vi "写入数据.vi"(7 "工作表名称":string="Sheet1", 8 "错误输入（无错误）":errorcluster, 9 "数据":variant, 10 "单元格区域":T2, 11 "引用簇":T1) -> (0 "错误输出":errorcluster, 3 "引用簇输出":T1)   [LabVIEW 2021, in "OperateExcel.lvlib"]
uses:
  OperateExcel.lvlib
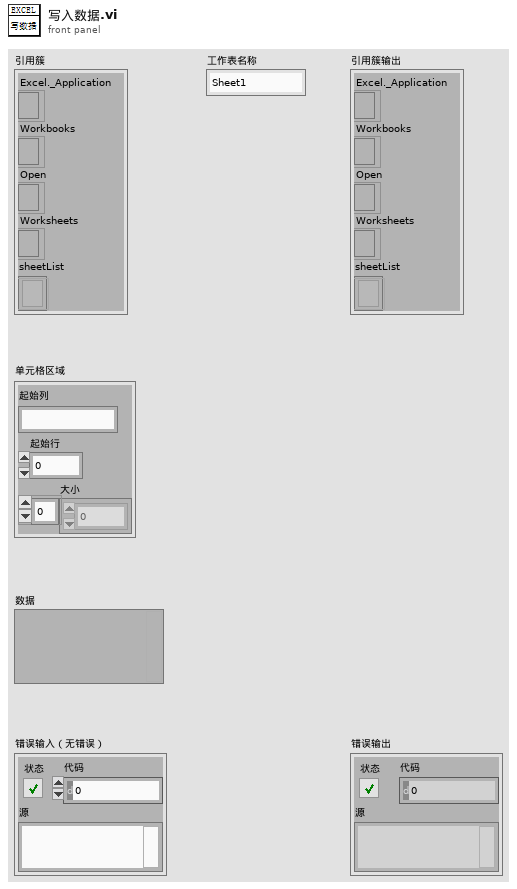
[diagram p1: front panel]
types:
  T1 = typedef "OperateExcel.lvlib/引用簇.ctl" = cluster{"Excel._Application":refnum<k7>, "Workbooks":refnum<k7>, "Open":refnum<k7>, "Worksheets":refnum<k7>, "sheetList":refnum<k7>[]}
  T2 = typedef "OperateExcel.lvlib/单元格区域.ctl" = cluster{"起始列":string, "起始行":i32, "大小":i32[]}
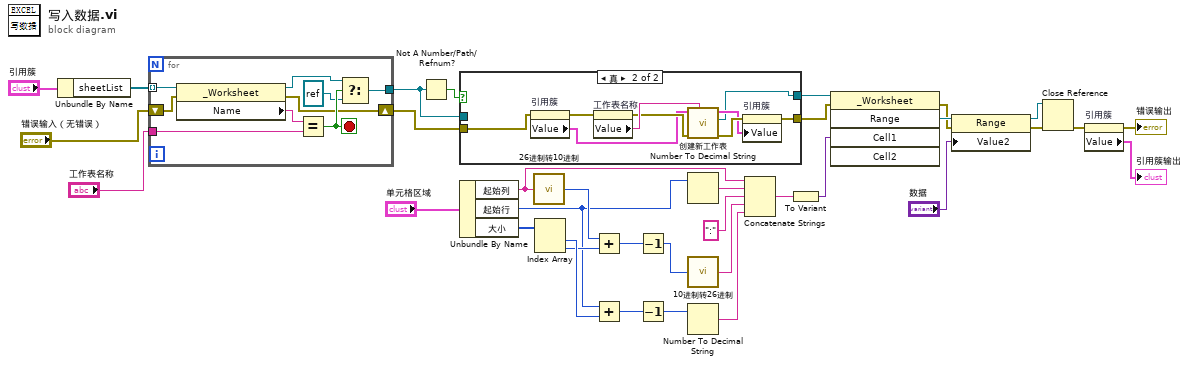
[diagram p0: block diagram]
diagram:
  n1 = Unbundle By Name("引用簇") -> ("sheetList"=w34:refnum<k7>[])
  n2 = for {
    tunnel: w34 -> [w43] mode=indexing
    tunnel: "工作表名称" -> [w41]
    tunnel: [w37] -> w31
    shift-right: [w35] -> w28
    shift-left: "错误输入（无错误）" -> [w36]
    stop <- w40 stop-if-true
    n3 = property class="_Worksheet"(reference=w43, error in=w36) -> (reference out=w38:refnum<k7>, error out=w35:errorcluster, "Name"=w42:string)
    n4 = Equal?(x=w42, y=w41) -> (x = y?=w40:bool)
    n5 = Select(t=w38, s=w40, f=refnum<k7> refnum ("自动化引用句柄")) -> (s? t:f=w37:refnum<k7>)
  }
  n6 = Not A Number/Path/Refnum?(number/path/refnum=w31) -> (NaN/Path/Refnum?=w32:bool)
  n7 = case shown="真" w32 {
    tunnel: w31 -> [w45 _]
    tunnel: [w45 w46] -> w30
    tunnel: w28 -> [w44 w52]
    tunnel: [w44 w48] -> w27
    frame False {
    }
    frame True {
      n8 = property on="引用簇" class="Clust (严格)"(error in=w52) -> (error out=w51:errorcluster, "Value"=w50:T1)  [unwired: 1 in, 1 out]
      n9 = property on="工作表名称" class="Str"(error in=w51) -> (error out=w53:errorcluster, "Value"=w54:string)  [unwired: 1 in, 1 out]
      n10 = call "创建新工作表.vi"("新工作表名称"=w54, "错误输入（无错误）"=w53, "引用簇"=w50) -> ("错误输出"=w49:errorcluster, "新工作表"=w46:refnum<k7>, "引用簇输出"=w47:T1)  [unwired: 5 in, 1 out]
      n11 = property on="引用簇" class="Clust (严格)"(error in=w49, "Value"=w47) -> (error out=w48:errorcluster)  [unwired: 1 in, 1 out]
    }
  }
  n12 = Unbundle By Name("单元格区域") -> ("起始列"=w13:string, "起始行"=w12:i32, "大小"=w19:i32[])
  n13 = call "26进制转10进制.vi"("26进制"=w13) -> ("十进制"=w15:i32)
  n14 = Index Array(array=w19) -> (element #1=w18:i32, element #2=w14:i32)  [unwired: 2 in]
  n15 = Add(x=w15, y=w14) -> (x+y=w16:i32)
  n16 = Add(x=w12, y=w18) -> (x+y=w17:i32)
  n17 = Decrement(x=w16) -> (x-1=w9:i32)
  n18 = Decrement(x=w17) -> (x-1=w7:i32)
  n19 = Number To Decimal String(number=w12) -> (decimal integer string=w11:string)  [unwired: 1 in]
  n20 = call "10进制转26进制.vi"("十进制"=w9) -> ("26进制"=w8:string)
  n21 = Number To Decimal String(number=w7) -> (decimal integer string=w6:string)  [unwired: 1 in]
  n22 = Concatenate Strings(w13, w11, ":" ("字符串"), w8, w6) -> (w5:string)
  n23 = To Variant(anything=w5) -> (Variant=w4:variant)
  n24 = invoke class="_Worksheet" method="Range"(reference=w30, error in=w27, "Cell1"=w4) -> (error out=w24:errorcluster, "Range"=w26:refnum<k7>)  [unwired: 2 in, 3 out]
  n25 = property class="Range"(reference=w26, error in=w24, "Value2"="数据") -> (reference out=w22:refnum<k7>, error out=w23:errorcluster)
  n26 = Close Reference(reference=w22, error in (no error)=w23) -> (error out=w3:errorcluster)
  n27 = property on="引用簇" class="Clust (严格)"(error in=w3) -> (error out=→"错误输出":errorcluster, "Value"=→"引用簇输出":T1)  [unwired: 1 in, 1 out]
